vi "Launch Digital Writer.vi"(8 "error in (no error)":errorcluster, 11 "Root Tester in":refnum<class "Root Tester.lvclass">) -> (0 "error out":errorcluster, 3 "Root Tester out":refnum<class "Root Tester.lvclass">)   [LabVIEW 2024, in "Root Tester.lvlib" / "Root Tester.lvclass"]
uses:
  Root Tester.lvclass
  C:/Program Files (x86)/National Instruments/LabVIEW 2024/vi.lib/ActorFramework/Actor/Actor.lvclass
  DAQmx Actor/Digital Writer/Digital Writer.lvclass
  DAQmx Actor/Digital Writer Messages/Digital Toggle Single Msg/Digital Toggle Single Msg.lvclass
  C:/Program Files (x86)/National Instruments/LabVIEW 2024/vi.lib/ActorFramework/Message/Message.lvclass
  Root Tester.lvclass/Root Tester.ctl
  <vilib>/DAQmx/create/channels.llb/DAQmx Create Channel (DO-Digital Output).vi
  <vilib>/ActorFramework/Actor/Actor.lvclass
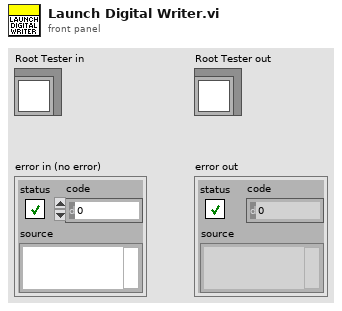
[diagram p1: front panel]
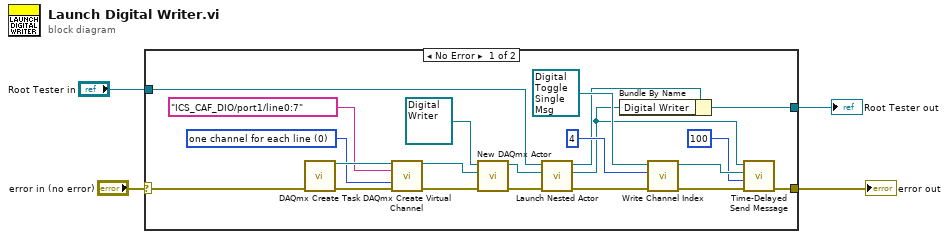
[diagram p0: block diagram]
diagram:
  n1 = case shown="No Error" "error in (no error)" {
    selector: "error in (no error)" -> [w21 w27]
    tunnel: [w8 w27] -> w3
    tunnel: [w5 w26] -> w1
    tunnel: "Root Tester in" -> [w17 w26]
    frame No Error {
      w18 = 0 items=["one channel for each line", "one channel for all lines"] ("line grouping")
      n2 = call <vilib>:"DAQmx Create Task.vi"("error in"=w21) -> ("task out"=w24:refnum<k21>, "error out"=w22:errorcluster)  [unwired: 13 in]
      n3 = call-poly <vilib>:"DAQmx Create Virtual Channel.vi"("task in"=w24, "lines"=tag "ICS_CAF_DIO/port1/line0:7", "line grouping"=w18, "error in"=w22) -> ("task out"=w19:refnum<k21>, "error out"=w20:errorcluster)  [unwired: 10 in]
      n4 = call-dynamic "New DAQmx Actor.vi"("error in (no error)"=w20, "DAQmx Task"=w19, "DAQmx Actor in"=refnum<class "Digital Writer.lvclass"> refnum ("DAQmx Actor.lvlib:Digital Writer.lvclass")) -> ("error out"=w15:errorcluster, "DAQmx Actor out"=w16:refnum<class "Digital Writer.lvclass">)  [unwired: 7 in]
      n5 = call <vilib>:"Launch Nested Actor.vi"("error in (no error)"=w15, "Nested Actor"=w16, "Caller Actor in"=w17) -> ("error out"=w11:errorcluster, "Nested Actor's Enqueuer"=w6:refnum<class "Message Enqueuer.lvclass">, "Caller Actor out"=w7:refnum<class "Root Tester.lvclass">)  [unwired: 6 in]
      n6 = Bundle By Name(cluster=w7, "Digital Writer"=w6) -> (w5:refnum<class "Root Tester.lvclass">)
      n7 = call-dynamic "Write Channel Index.vi"("error in (no error)"=w11, "Channel Index"=4, "Digital Toggle Single Msg in"=refnum<class "Digital Toggle Single Msg.lvclass"> refnum) -> ("error out"=w10:errorcluster, "Digital Toggle Single Msg out"=w14:refnum<class "Digital Toggle Single Msg.lvclass">)  [unwired: 7 in]
      n8 = call <vilib>:"Time-Delayed Send Message.vi"("error in (no error)"=w10, "Milliseconds To Wait"=100, "Message"=w14, "Message Enqueuer"=w6) -> ("error out"=w8:errorcluster)  [unwired: 6 in, 1 out]
    }
    frame Error {
    }
  }
  "error out" <- w3
  "Root Tester out" <- w1
